vi "Calculate effective field of view from coord list params.vi"() -> (3 "Effective FOV (um)":sgl)   [LabVIEW 2020]
uses:
  User Interface/Windows/Coordinates list window/Globals/Coord window-Globals.vi
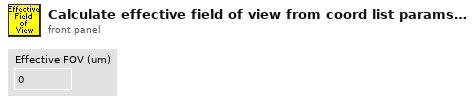
[diagram p1: front panel]
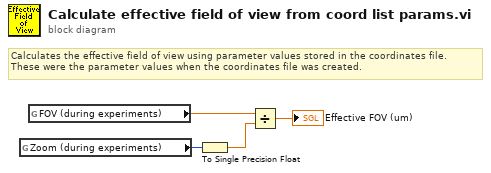
[diagram p0: block diagram]
diagram:
  # "Calculates the effective field of view using parameter values stored in the coordinates file.\nThese were the parameter values when the coordinates file was created."
  n1 = global read "Coord window-Globals.vi" "Zoom (during experiments)"() -> (w1:i8)
  n2 = global read "Coord window-Globals.vi" "FOV (during experiments)"() -> (w2:sgl)
  n3 = To Single Precision Float(number=w1) -> (single precision float=w4:sgl)
  n4 = Divide(x=w2, y=w4) -> (x/y=→"Effective FOV (um)":sgl)
